vi "myRIO_BRig_RT_comm_webdav_uploadReceived_main.vi"(10 "input_dataSize":i32, 11 "input_dataName":string="dataExp") -> ()   [LabVIEW 2014]
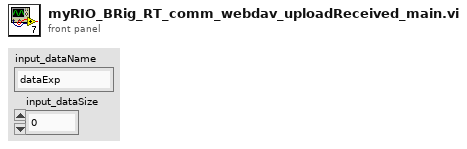
[diagram p1: front panel]
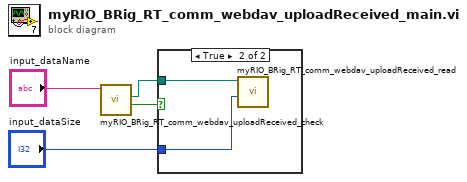
[diagram p0: block diagram]
diagram:
  n1 = call "myRIO_BRig_RT_comm_webdav_uploadReceived_check.vi"("input_dataName"="input_dataName") -> ("output_Iexist"=w4:bool, "output_dataPath"=w3:path)  [unwired: 9 in]
  n2 = case shown="True" w4 {
    tunnel: w3 -> [_ w6]
    tunnel: "input_dataSize" -> [_ w5]
    frame False {
    }
    frame True {
      n3 = call "myRIO_BRig_RT_comm_webdav_uploadReceived_read.vi"("input_dataSize"=w5, "input_filePath"=w6) -> ()  [unwired: 8 in, 2 out]
    }
  }
